vi "PicoScope3000aNearestSampleInterval.vi"(5 "Enabled array":i16[](array[numeric])=[0, 0, 0, 0, 0, 0, 0, 0, 0, 0], 6 "Acquisition Settings":T1 {"postTriggerSamples" format="%_6p"; "preTriggerSamples" format="%_6p"}, 8 "error in (no error)":errorcluster, 9 "roundFaster":bool, 10 "timeIntervalRequested":dbl format="%#6_6p", 11 "handle in":i16) -> (0 "error out":errorcluster, 1 "timebase":u32, 2 "timeIntervalAvailable":dbl format="%#6_6p", 3 "handle out":i16)   [LabVIEW 2010]
doc: "Calls Gettimebase function"
uses:
  ps3000a.dll
  shared/Acquisition Settings.ctl
panel:
  in  "Memory Segment":u32
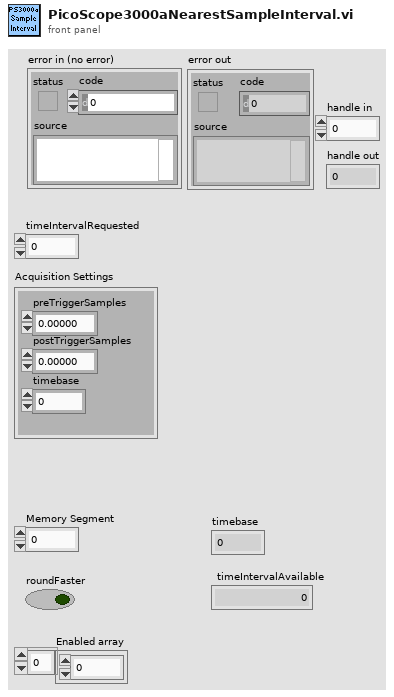
[diagram p1: front panel]
types:
  T1 = typedef "Acquisition Settings.ctl" = cluster{"preTriggerSamples":u64, "postTriggerSamples":u64, "timebase":u32}
  T2 = cluster{"status":bool, "code":u32, "source":string}
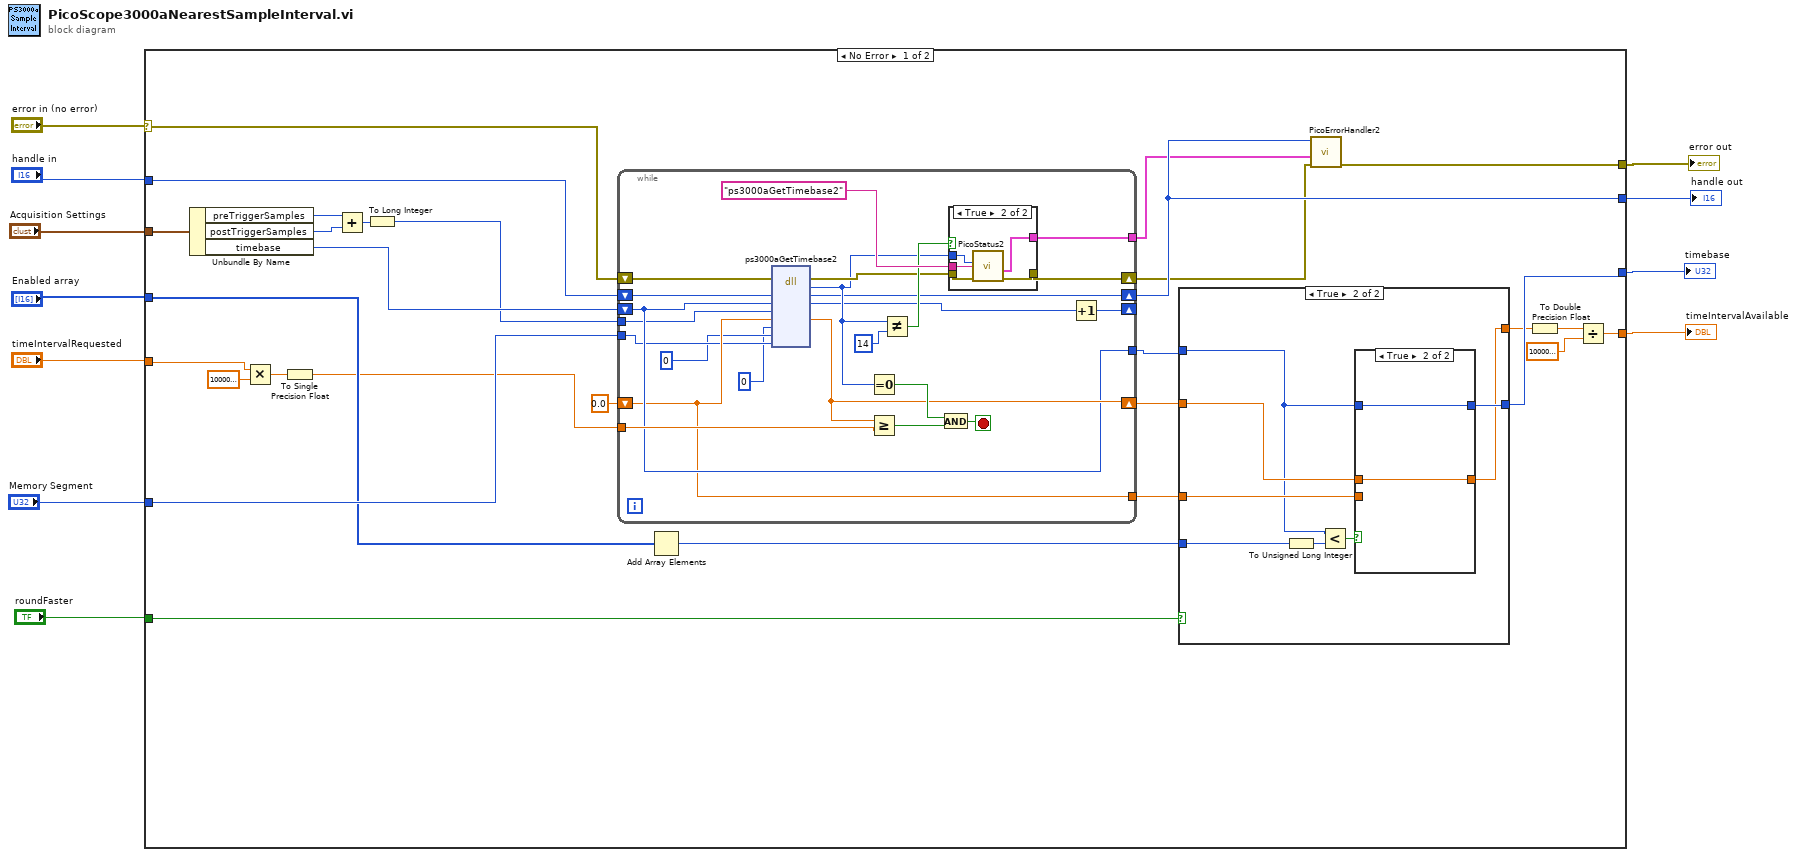
[diagram p0: block diagram]
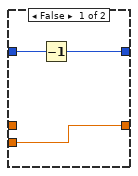
[diagram p3: hidden frame]
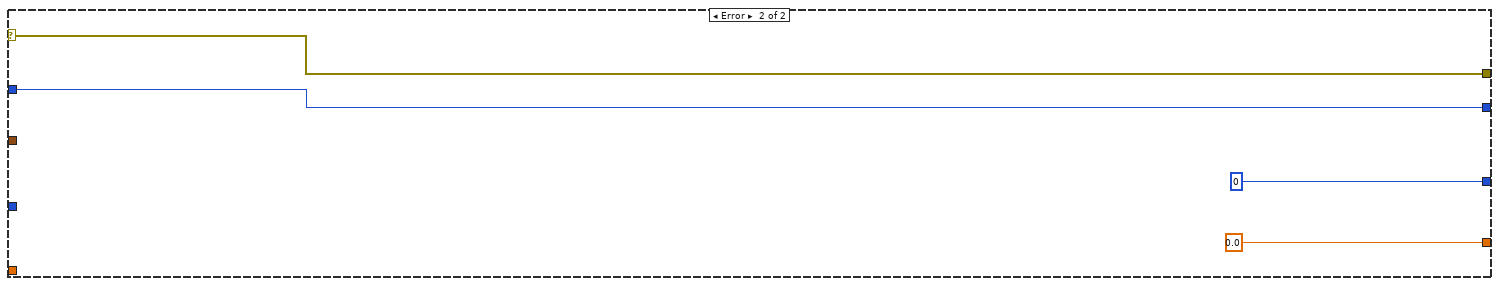
[diagram p5: hidden frame]
diagram:
  n1 = case shown="No Error" "error in (no error)" {
    selector: "error in (no error)" -> [w18 w88]
    tunnel: [w40 w88] -> w11
    tunnel: [w31 w87] -> w10
    tunnel: "handle in" -> [w32 w87]
    tunnel: "Enabled array" -> [w20 _]
    tunnel: "roundFaster" -> [w24 _]
    tunnel: "timeIntervalRequested" -> [w37 _]
    tunnel: [w21 u32 0 ("timebase")] -> w4
    tunnel: [w28 0.0 ("timeIntervalAvailable")] -> w3
    tunnel: "Acquisition Settings" -> [w33 _]
    tunnel: "Memory Segment" -> [w30 _]
    frame No Error {
      n2 = Unbundle By Name(w33) -> ("preTriggerSamples"=w35:u64, "postTriggerSamples"=w36:u64, "timebase"=w25:u32)
      n3 = Multiply(x=w37, y=1000000000.0) -> (x*y=w38:dbl)
      n4 = To Single Precision Float(number=w38) -> (single precision float=w17:sgl)
      n5 = Add(x=w35, y=w36) -> (x+y=w34:u64)
      n6 = To Long Integer(number=w34) -> (32bit integer=w19:i32)
      n7 = while {
        tunnel: w19 -> [w60]
        tunnel: w30 -> [w58]
        shift-right: [w66] -> w31
        shift-left: w32 -> [w62]
        shift-right: [w78] -> w27
        shift-left: w18 -> [w63]
        tunnel: [w76] -> w26
        shift-right: [w75] -> _
        shift-left: w25 -> [w61]
        tunnel: w17 -> [w74]
        shift-right: [w64] -> w22
        shift-left: sgl 0.0 ("timeIntervalNanoseconds") -> [w59]
        tunnel: [w59] -> w23
        tunnel: [w61] -> w13
        stop <- w73 stop-if-true
        n8 = dll-call lib="ps3000a.dll" fn="ps3000aGetTimebase2"(error in=w63, "handle"=w62, "timebase"=w61, "noSamples"=w60, "timeIntervalNanoseconds"=w59, "oversample"=i16 0, "maxSamples"=0, "segmentIndex"=w58) -> (error out=w68:errorcluster, "PICO_STATUS"=w67:u32, "handle"=w66:i16, "timebase"=w65:u32, "timeIntervalNanoseconds"=w64:sgl)  [unwired: 6 in, 1 out]
        n9 = Equal To 0?(x=w67) -> (x = 0?=w71:bool)
        n10 = Greater Or Equal?(x=w64, y=w74) -> (x >= y?=w72:bool)
        n11 = Not Equal?(x=w67, y=u32 14) -> (x != y?=w69:bool)
        n12 = And(x=w71, y=w72) -> (x .and. y?=w73:bool)
        n13 = case shown="True" w69 {
          tunnel: w68 -> [w79 w84]
          tunnel: [w79 w83] -> w78
          tunnel: "ps3000aGetTimebase2" ("source") -> [_ w82]
          tunnel: [_ w81] -> w76
          tunnel: w67 -> [_ w80]
          frame False {
          }
          frame True {
            n14 = call "PicoStatus2.vi"("PICO source"=w82, "Error in"=w84, "PICO STATUS"=w80) -> ("error out"=w83:errorcluster, "PICO_STATUS out"=w81:T2)  [unwired: 5 in]
          }
        }
        n15 = Increment(x=w65) -> (x+1=w75:u32)
      }
      n16 = Add Array Elements(numeric array=w20) -> (sum=w12:i16)
      n17 = case shown="True" w24 {
        tunnel: [w42 w49] -> w14
        tunnel: w23 -> [_ w48]
        tunnel: w22 -> [w42 w47]
        tunnel: [w41 w50] -> w21
        tunnel: w13 -> [w41 w45]
        tunnel: w12 -> [_ w43]
        frame False {
        }
        frame True {
          n18 = To Unsigned Long Integer(number=w43) -> (unsigned 32bit integer=w44:u32)
          n19 = Less?(x=w45, y=w44) -> (x < y?=w46:bool)
          n20 = case shown="True" w46 {
            tunnel: [w53 w55] -> w50
            tunnel: w45 -> [w52 w55]
            tunnel: [w51 w54] -> w49
            tunnel: w48 -> [w51 _]
            tunnel: w47 -> [_ w54]
            frame False {
              n21 = Decrement(x=w52) -> (x-1=w53:u32)
            }
            frame True {
            }
          }
        }
      }
      n22 = call "PicoErrorHandler2.vi"("error in (no error)"=w27, "PICO_STATUS in"=w26, "handle In"=w31) -> ("error out"=w40:errorcluster)  [unwired: 8 in]
      n23 = To Double Precision Float(number=w14) -> (double precision float=w15:dbl)
      n24 = Divide(x=w15, y=1000000000.0) -> (x/y=w28:dbl)
    }
    frame Error {
    }
  }
  "error out" <- w11
  "handle out" <- w10
  "timebase" <- w4
  "timeIntervalAvailable" <- w3
